vi "Read Key (U32).vi"(7 "section":string caption="Abschnitt", 8 "error in (no error)":errorcluster caption="Fehler (Eingang, kein Fehler)", 9 "default value":u32 caption="Standardwert", 10 "key":string caption="Schlüssel", 11 "refnum":T1 caption="RefNum") -> (0 "error out":errorcluster caption="Fehler (Ausgang)", 1 "value":u32 caption="Wert", 2 "found?":bool caption="Gefunden?", 3 "refnum out":T1 caption="RefNum (Ausgang)")   [LabVIEW 2009]
doc: "Liest einen Wert, der einem Schlüssel in einem angegebenen Abschnitt in der durch <B>Refnum</B> angegebenen Konfigurationsdatei zugeordnet ist. Wenn der Schlüssel nicht existiert, wird vom VI der Standardwert ausgegeben. Mit diesem polymorphen VI können folgende Wertetypen aus einem Schlüssel ausgelesen werden: boolesche Werte, numerische Werte mit doppelter Genauigkeit, vorzeichenbehaftete Integer-Werte, Pfade, Strings und vorzeichenlose Integer-Werte. Durch den Datentyp, der am Eingang <B>Index</B> anliegt, wird die zu verwendende Instanz des polymorphen VIs festgelegt."
uses:
  <vilib>/Utility/config.llb/Config Data RefNum.ctl
  <vilib>/Utility/config.llb/NI_LVConfig.lvlib
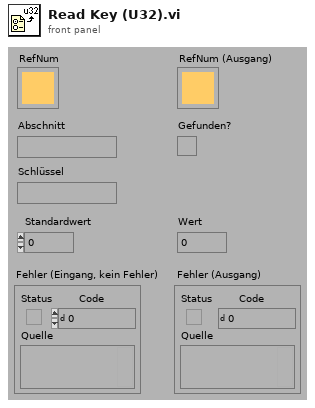
[diagram p1: front panel]
types:
  T1 = typedef "NI_LVConfig.lvlib/Config Data RefNum.ctl" = refnum<k1>
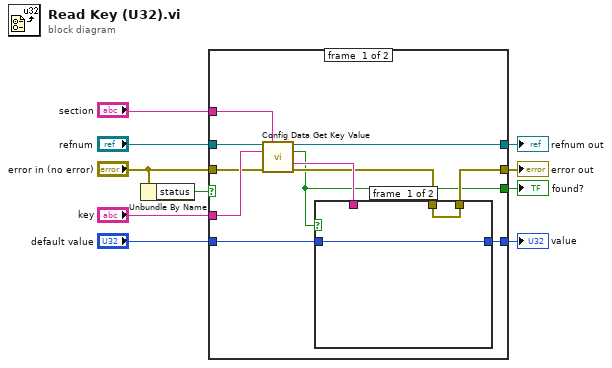
[diagram p0: block diagram]
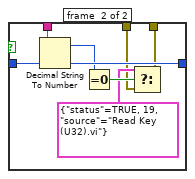
[diagram p2: hidden frame]
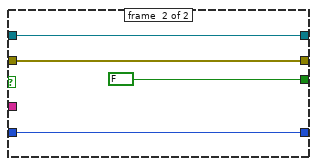
[diagram p3: hidden frame]
diagram:
  n1 = Unbundle By Name("error in (no error)") -> ("status"=w10:bool)
  n2 = case shown="False" w10 {
    tunnel: [w18 w34] -> w1
    tunnel: [w12 w35] -> w2
    tunnel: "refnum" -> [w14 w34]
    tunnel: "error in (no error)" -> [w15 w35]
    tunnel: "section" -> [w21 _]
    tunnel: "key" -> [w20 _]
    tunnel: [w11 FALSE ("section exists?")] -> w4
    tunnel: [w19 w33] -> w3
    tunnel: "default value" -> [w16 w33]
    frame #0 {
      n3 = call "Config Data Get Key Value.vi"("config data"=w14, "section"=w21, "key"=w20, "error in (no error)"=w15) -> ("config data out"=w18:T1, "key exists?"=w11:bool, "key value"=w17:string, "error out"=w13:errorcluster)  [unwired: 6 in, 2 out]
      n4 = case shown="True" w11 {
        tunnel: [w22 w31] -> w19
        tunnel: w17 -> [_ w30]
        tunnel: w16 -> [w22 w29]
        tunnel: w13 -> [w23 w25]
        tunnel: [w23 w24] -> w12
        frame #0 {
        }
        frame #1 {
          n5 = Decimal String To Number(string=w30, default (0L)=w29) -> (offset past number=w26:i32, number=w31:u32)  [unwired: 1 in]
          n6 = Equal To 0?(x=w26) -> (x = 0?=w28:bool)
          n7 = Select(t=cluster{"status":bool, u16, "source":string} {"status"=TRUE, 19, "source"="Read Key (U32).vi"} ("f"), s=w28, f=w25) -> (s? t:f=w24:errorcluster)
        }
      }
    }
    frame #1 {
    }
  }
  "error out" <- w2
  "refnum out" <- w1
  "value" <- w3
  "found?" <- w4
